vi "Clear Subpanel.vi"(8 "error in (no error)":errorcluster, 11 "Protected Subpanel":T1) -> (0 "error out":errorcluster, 3 "Protected Subpanel Out":T1)   [LabVIEW 2020, in "MVA Framework.lvlib" / "IViewable.lvlib" / "ProtectedSubpanel.lvclass"]
doc: "清除子面板"
uses:
  ProtectedSubpanel.lvclass
  Protected Subpanel Reference.ctl
  ProtectedSubpanel.lvclass/ProtectedSubpanel.ctl
  <vilib>/ActorFramework/Message Enqueuer/Message Enqueuer.lvclass
  <vilib>/ActorFramework/Message Enqueuer/Message Enqueuer.lvclass/Message Enqueuer.ctl
  <vilib>/ActorFramework/Message Enqueuer/Enqueue.vi
  IViewable Messages/Removed From Subpanel Msg/Removed From Subpanel Msg.lvclass
  C:/Program Files/National Instruments/LabVIEW 2020/vi.lib/ActorFramework/Message/Message.lvclass
  <vilib>/ActorFramework/Message Priority Queue/Priority Enqueue.vi
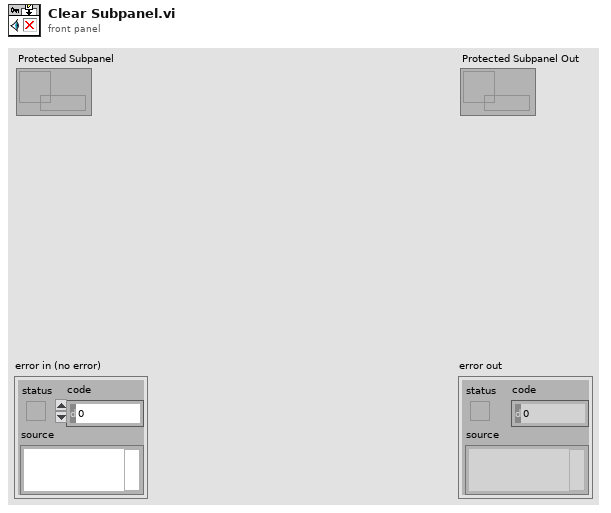
[diagram p1: front panel]
types:
  T1 = typedef "MVA Framework.lvlib/IViewable.lvlib/ProtectedSubpanel.lvclass/Protected Subpanel Reference.ctl" = refnum<data-value>
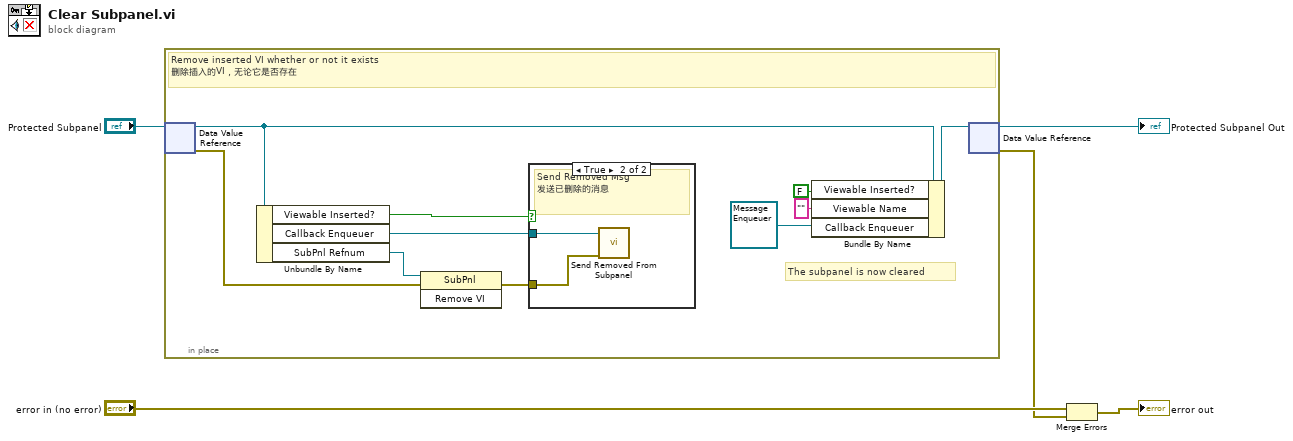
[diagram p0: block diagram]
diagram:
  n1 = in-place {
    # "The subpanel is now cleared"
    # "Remove inserted VI whether or not it exists\n删除插入的VI，无论它是否存在"
    n2 = in-place-dvr #1("Protected Subpanel") -> (w15:refnum<class "ProtectedSubpanel.lvclass">, w13:errorcluster)
    n3 = Unbundle By Name(w15) -> ("Viewable Inserted?"=w6:bool, "Callback Enqueuer"=w8:refnum<class "Message Enqueuer.lvclass">, "SubPnl Refnum"=w14:refnum<vi>)
    n4 = invoke class="SubPnl" method="Remove VI"(reference=w14, error in=w13) -> (error out=w7:errorcluster)  [unwired: 1 in, 2 out]
    n5 = case shown="True" w6 {
      tunnel: w8 -> [_ w17]
      tunnel: w7 -> [_ w16]
      frame False {
        # "Nothing inserted"
      }
      frame True {
        # "Send Removed Msg\n发送已删除的消息"
        n6 = call "Send Removed From Subpanel.vi"("error in (no error)"=w16, "Message Enqueuer"=w17) -> ()  [unwired: 8 in, 2 out]
      }
    }
    n7 = Bundle By Name(cluster=w15, "Viewable Inserted?"=FALSE, "Viewable Name"="", "Callback Enqueuer"=refnum<class "Message Enqueuer.lvclass"> refnum) -> (w12:refnum<class "ProtectedSubpanel.lvclass">)
    n8 = in-place-dvr #1(w12) -> (→"Protected Subpanel Out":T1, w1:errorcluster)
  }
  n9 = Merge Errors("error in (no error)", w1) -> (→"error out":errorcluster)
